vi "create log file.vi"(8 "error in (no error)":errorcluster, 11 "Socket in":refnum<class "Socket.lvclass">) -> (0 "error out":errorcluster, 3 "Socket out":refnum<class "Socket.lvclass">)   [LabVIEW 2018, in "Socket.lvclass"]
uses:
  Socket.lvclass
  Socket.lvclass/Socket.ctl
  Log File/CM_Log File.lvclass/CM_Log File.ctl
  Log File/CM_Log File.lvclass
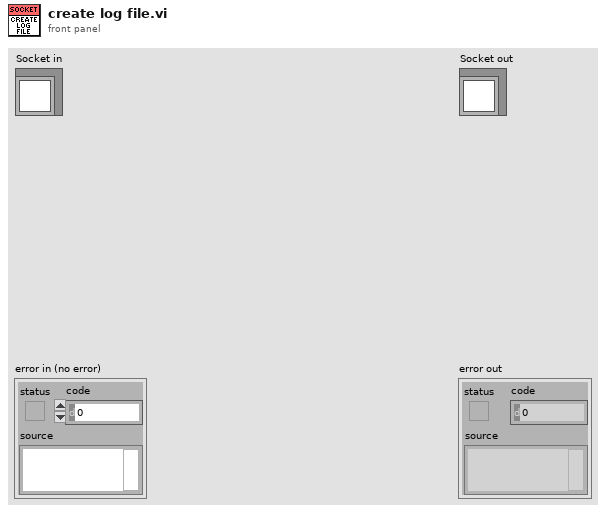
[diagram p1: front panel]
types:
  T1 = typedef "LVDateTimeRec.ctl" = cluster{"fractional second":dbl, "second":i32, "minute":i32, "hour":i32, "day of month":i32, "month":i32, "year":i32, "day of week":i32, "day of year":i32, "DST":i32}
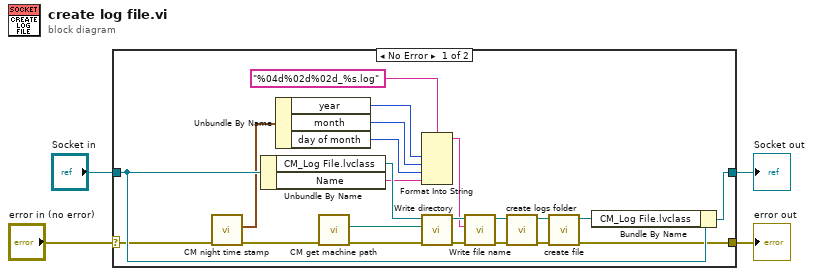
[diagram p0: block diagram]
diagram:
  n1 = case shown="No Error" "error in (no error)" {
    selector: "error in (no error)" -> [w13 w28]
    tunnel: [w18 w28] -> w3
    tunnel: [w22 w27] -> w1
    tunnel: "Socket in" -> [w23 w27]
    frame No Error {
      n2 = call "CM night time stamp.vi"("error in (no error)"=w13) -> ("error out"=w12:errorcluster, "date time rec"=w7:T1)  [unwired: 9 in]
      n3 = Unbundle By Name(w23) -> ("CM_Log File.lvclass"=w26:refnum<class "CM_Log File.lvclass">, "Name"=w5:string)
      n4 = Unbundle By Name(w7) -> ("year"=w11:i32, "month"=w10:i32, "day of month"=w9:i32)
      n5 = call "CM get machine path.vi"("error in (no error) 2"=w12) -> ("error in (no error)"=w25:errorcluster, "machine path"=w24:path)  [unwired: 9 in]
      n6 = Format Into String(format string="%04d%02d%02d_%s.log", w11, w10, w9, w5) -> (resulting string=w6:string)  [unwired: 2 in, 1 out]
      n7 = call "Write directory.vi"("error in (no error)"=w25, "directory"=w24, "Log File in"=w26) -> ("error out"=w15:errorcluster, "Log File out"=w17:refnum<class "CM_Log File.lvclass">)  [unwired: 7 in]
      n8 = call "Write file name.vi"("error in (no error)"=w15, "file name"=w6, "Log File in"=w17) -> ("error out"=w14:errorcluster, "Log File out"=w16:refnum<class "CM_Log File.lvclass">)  [unwired: 7 in]
      n9 = call "create logs folder.vi"("error in (no error)"=w14, "Log File in"=w16) -> ("error out"=w19:errorcluster, "Log File out"=w21:refnum<class "CM_Log File.lvclass">)  [unwired: 8 in]
      n10 = call "create file.vi"("error in (no error)"=w19, "Log File in"=w21) -> ("error out"=w18:errorcluster, "Log File out"=w20:refnum<class "CM_Log File.lvclass">)  [unwired: 8 in]
      n11 = Bundle By Name(cluster=w23, "CM_Log File.lvclass"=w20) -> (w22:refnum<class "Socket.lvclass">)
    }
    frame Error {
    }
  }
  "error out" <- w3
  "Socket out" <- w1
